vi "Raw Data.vi"() -> ()   [LabVIEW 2016, in "Drive System.lvlib"]
uses:
  Drive System.lvlib
panel:
  in  "Locking VI":string
  out "Locked?":bool
  in  "SP R":dbl
  in  "SP L":dbl
  in  "Motor R":dbl
  in  "Motor L":dbl
  in  "Encoder R":dbl
  in  "Encoder L":dbl
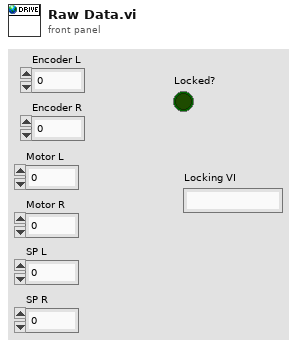
[diagram p1: front panel]
diagram:
